vi "StartSequenceAcquisition1.vi"(0 "Camera_Prime95B in":refnum<class "Camera_Prime95B.lvclass">, 5 "DataExchange":T1, 11 "error in (no error)":errorcluster) -> (4 "Camera_Prime95B out":refnum<class "Camera_Prime95B.lvclass">, 15 "error out":errorcluster)   [LabVIEW 2020]
uses:
  E:/Development/DevHardSoftware/MicroscopyFramework/Model/Hardware Layer/Real Hardware/Camera_Prime95B/Camera_Prime95B/Dependencies/PVCamNET.dll
  Dependencies/PVCamNET.dll
  Wait For Stop Status.ctl
  Camera_Prime95B.lvclass
  Camera Status.ctl
  Acquisition Params.ctl
  Hardware Abstraction Layer/Component/Device/Device/DeviceStatus.ctl
  Hardware Abstraction Layer/Component/Device/Device.lvlib
  E:/Development/DevHardSoftware/MicroscopyFramework/Model/Hardware Abstraction Layer/Component/Camera/Camera/Camera.lvclass
  E:/Development/DevHardSoftware/MicroscopyFramework/Model/Hardware Abstraction Layer/Component/Device/Device/Device.lvclass
  C:/Program Files/National Instruments/LabVIEW 2020/vi.lib/ActorFramework/Actor/Actor.lvclass
  E:/Development/DevHardSoftware/MicroscopyFramework/Model/Hardware Layer/Real Hardware/Camera_Prime95B/Camera_Prime95B/Camera_Prime95B.lvclass
  Hardware Abstraction Layer/Component/Device/Device/DataExchange.ctl
  Interface/DataListener/DataListener.lvclass
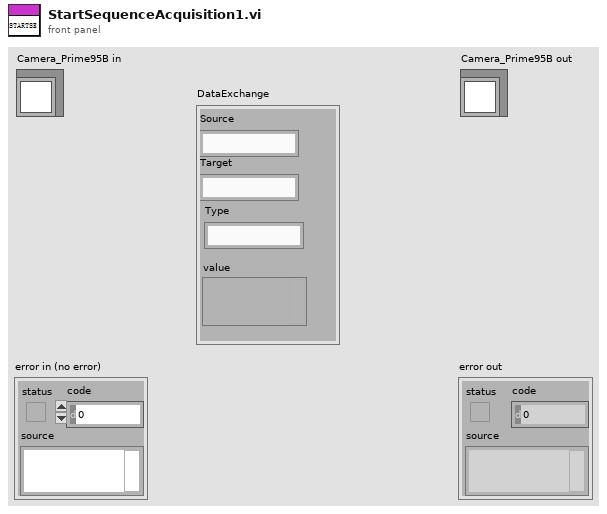
[diagram p1: front panel]
types:
  T1 = typedef "DataListener.lvclass/DataExchange.ctl" = cluster{"Source":string, "Target":string, "Type":string, "value":variant}
  T2 = typedef "Camera_Prime95B.lvlib/Camera_Prime95B.lvclass/Acquisition Params.ctl" = cluster{"ExposureMs":dbl, "Frames":dbl, "Interval":dbl, "Save Path":path, "Stream Save Path":path, "SingleStack?":bool, "StreamToDisk?":bool, "Alert when finish?":bool, "File suffix":string}
  T3 = typedef "Device.lvlib/DeviceStatus.ctl" = i32
  T4 = typedef "Camera_Prime95B.lvlib/Camera_Prime95B.lvclass/Wait For Stop Status.ctl" = i32
  T5 = typedef "Camera_Prime95B.lvlib/Camera_Prime95B.lvclass/Camera Status.ctl" = i32
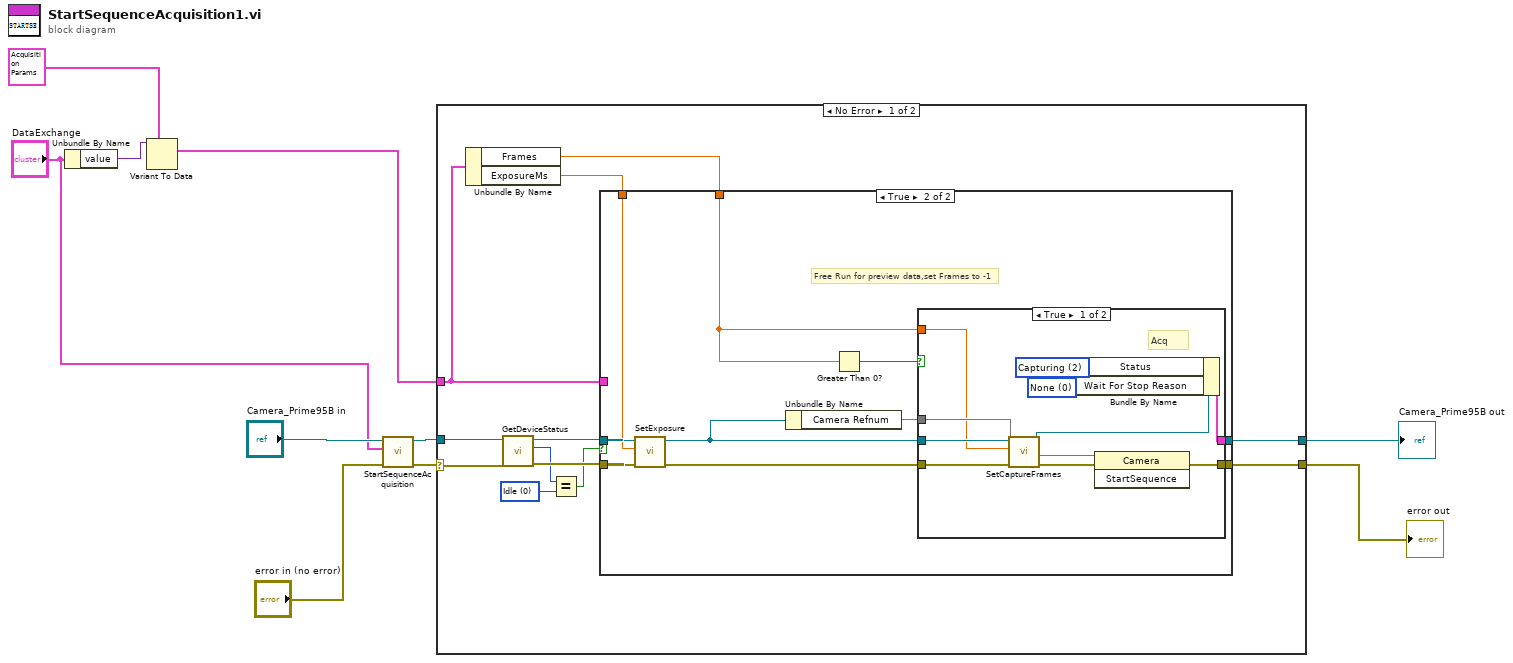
[diagram p0: block diagram]
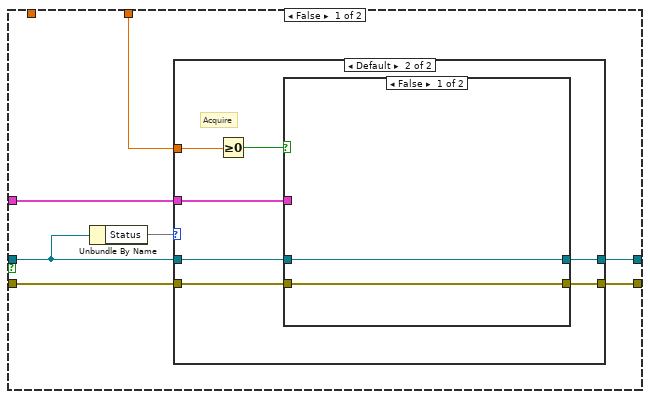
[diagram p2: hidden frame]
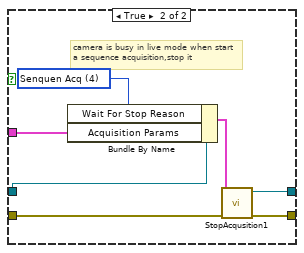
[diagram p4: hidden frame]
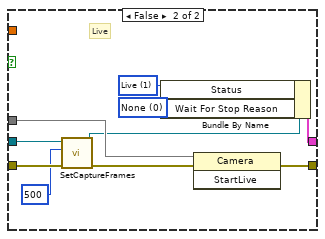
[diagram p5: hidden frame]
diagram:
  n1 = Unbundle By Name("DataExchange") -> ("value"=w4:variant)
  n2 = Variant To Data(type=T2 {"ExposureMs"=0.0, "Frames"=0.0, "Interval"=0.0, "Save Path"=path "", "Stream Save Path"=path "", "SingleStack?"=FALSE, "StreamToDisk?"=FALSE, "Alert when finish?"=FALSE, "File suffix"=""} ("Acquisition Params"), Variant=w4) -> (data=w1:T2)  [unwired: 1 in, 1 out]
  n3 = call-dynamic "StartSequenceAcquisition.vi"("error in (no error)"="error in (no error)", "DataExchange"="DataExchange", "Camera_Prime95B in"="Camera_Prime95B in") -> ("error out"=w9:errorcluster, "Camera_Prime95B out"=w10:refnum<class "Camera_Prime95B.lvclass">)  [unwired: 7 in]
  n4 = case shown="No Error" w9 {
    selector: w9 -> [w22 w79]
    tunnel: [w19 w79] -> w5
    tunnel: w10 -> [w21 w78]
    tunnel: [w20 w78] -> w6
    tunnel: w1 -> [w13 _]
    frame No Error {
      w15 = T3 0 items=["Idle", "Busy"] ("y")
      n5 = Unbundle By Name(w13) -> ("Frames"=w11:dbl, "ExposureMs"=w12:dbl)
      n6 = call-dynamic "GetDeviceStatus.vi"("error in (no error)"=w22, "Camera_Prime95B in"=w21) -> ("error out"=w17:errorcluster, "Status"=w16:T3, "Camera_Prime95B out"=w18:refnum<class "Camera_Prime95B.lvclass">)  [unwired: 7 in]
      n7 = Equal?(x=w16, y=w15) -> (x = y?=w14:bool)
      n8 = case shown="True" w14 {
        tunnel: w18 -> [w28 w51]
        tunnel: [w27 w49] -> w20
        tunnel: [w25 w57] -> w19
        tunnel: w11 -> [w24 w48]
        tunnel: w12 -> [_ w56]
        tunnel: w17 -> [w26 w50]
        tunnel: w13 -> [w23 _]
        frame False {
          n9 = Unbundle By Name(w28) -> ("Status"=w29)
          n10 = case shown="Default" w29 {
            tunnel: w28 -> [w31 w36]
            tunnel: [w31 w35] -> w27
            tunnel: w26 -> [w30 w38]
            tunnel: [w30 w37] -> w25
            tunnel: w24 -> [_ w34]
            tunnel: w23 -> [_ w32]
            frame 2 {
              # "Is in Acquiring"
            }
            frame Default {
              # "Acquire"
              n11 = Greater Or Equal To 0?(x=w34) -> (x >= 0?=w33:bool)
              n12 = case shown="False" w33 {
                tunnel: w38 -> [w39 w47]
                tunnel: [w39 w46] -> w37
                tunnel: w36 -> [w40 w44]
                tunnel: [w40 w42] -> w35
                tunnel: w32 -> [_ w41]
                frame False {
                }
                frame True {
                  w45 = T4 4 items=["None", "Set Exposure", "Set Binning", "Set ROI", "Senquen Acq", ""] ("Wait For Stop Reason")
                  # "camera is busy in live mode when start\na sequence acquisition,stop it"
                  n13 = Bundle By Name(cluster=w44, "Wait For Stop Reason"=w45, "Acquisition Params"=w41) -> (w43:cluster{})
                  n14 = call-dynamic "StopAcqusition1.vi"("error in (no error)"=w47, "Camera_Prime95B in"=w43) -> ("error out"=w46:errorcluster, "Camera_Prime95B out"=w42:refnum<class "Camera_Prime95B.lvclass">)  [unwired: 8 in]
                }
              }
            }
          }
        }
        frame True {
          # "Free Run for preview data,set Frames to -1"
          n15 = call-dynamic "SetExposure.vi"("error in (no error)"=w50, "Setting.Exposure"=w56, "Camera_Prime95B in"=w51) -> ("error out"=w54:errorcluster, "Camera_Prime95B out"=w55:refnum<class "Camera_Prime95B.lvclass">)  [unwired: 7 in]
          n16 = Unbundle By Name(w55) -> ("Camera Refnum"=w53)
          n17 = Greater Than 0?(x=w48) -> (x > 0?=w52:bool)
          n18 = case shown="True" w52 {
            tunnel: [w67 w77] -> w57
            tunnel: w54 -> [w65 w75]
            tunnel: w53 -> [w66 w76]
            tunnel: w55 -> [w64 w73]
            tunnel: [w60 w70] -> w49
            tunnel: w48 -> [w61 _]
            frame True {
              w58 = T4 0 items=["None", "Set Exposure", "Set Binning", "Set ROI", "Senquen Acq", ""] ("Wait For Stop Reason")
              w59 = T5 2 items=["Idle", "Live", "Capturing"] ("Status")
              # "Acq"
              n19 = call-dynamic "SetCaptureFrames.vi"("error in (no error)"=w65, "Setting.FramesToCapture"=w61, "Camera_Prime95B in"=w64) -> ("error out"=w62:errorcluster, "Camera_Prime95B out"=w63:refnum<class "Camera_Prime95B.lvclass">)  [unwired: 7 in]
              n20 = Bundle By Name(cluster=w63, "Status"=w59, "Wait For Stop Reason"=w58) -> (w60:cluster{})
              n21 = invoke class="Camera" method="StartSequence"(reference=w66, error in=w62) -> (error out=w67:errorcluster)  [unwired: 1 in, 2 out]
            }
            frame False {
              w68 = T4 0 items=["None", "Set Exposure", "Set Binning", "Set ROI", "Senquen Acq", ""] ("Wait For Stop Reason")
              w69 = T5 1 items=["Idle", "Live", "Capturing"] ("Status")
              # "Live"
              n22 = call-dynamic "SetCaptureFrames.vi"("error in (no error)"=w75, "Setting.FramesToCapture"=500, "Camera_Prime95B in"=w73) -> ("error out"=w74:errorcluster, "Camera_Prime95B out"=w71:refnum<class "Camera_Prime95B.lvclass">)  [unwired: 7 in]
              n23 = Bundle By Name(cluster=w71, "Status"=w69, "Wait For Stop Reason"=w68) -> (w70:cluster{})
              n24 = invoke class="Camera" method="StartLive"(reference=w76, error in=w74) -> (error out=w77:errorcluster)  [unwired: 1 in, 2 out]
            }
          }
        }
      }
    }
    frame Error {
    }
  }
  "error out" <- w5
  "Camera_Prime95B out" <- w6
